vi "array_to_pixmap.vi"(11 "photoarray":u32[][](array[numeric])) -> (2 "pixmap out":T1, 3 "photoarray out":u32[][](array[numeric]))   [LabVIEW 2016]
uses:
  <vilib>/picture/picture.llb/imagedata.ctl
panel:
  out "new picture":picture
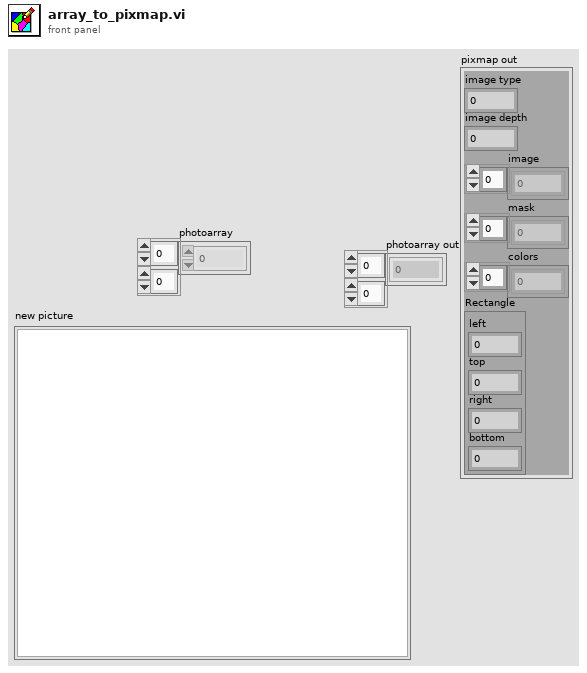
[diagram p1: front panel]
types:
  T1 = typedef "imagedata.ctl" = cluster{"image type":i32, "image depth":i32, "image":u8[], "mask":u8[], "colors":u32[], "Rectangle":cluster{"left":i16, "top":i16, "right":i16, "bottom":i16}}
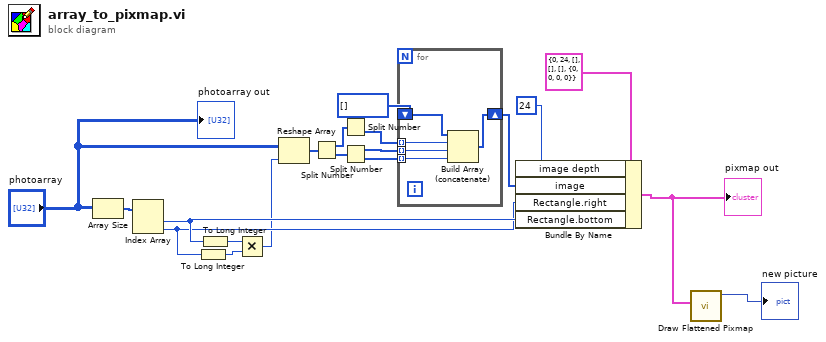
[diagram p0: block diagram]
diagram:
  n1 = Array Size(array="photoarray") -> (size(s)=w19:i32[])
  n2 = Index Array(array=w19) -> (element #1=w17:i32, element #2=w16:i32)  [unwired: 2 in]
  n3 = To Long Integer(number=w16) -> (32bit integer=w13:i32)
  n4 = To Long Integer(number=w17) -> (32bit integer=w14:i32)
  n5 = Multiply(x=w14, y=w13) -> (x*y=w12:i32)
  n6 = Reshape Array("photoarray", w12) -> (w11:u32[])
  n7 = Split Number(x=w11) -> (hi(x)=w10:u16[], lo(x)=w9:u16[])
  n8 = Split Number(x=w10) -> (lo(x)=w3:u8[])  [unwired: 1 out]
  n9 = Split Number(x=w9) -> (hi(x)=w4:u8[], lo(x)=w5:u8[])
  n10 = for {
    shift-right: [w24] -> w8
    shift-left: u8[] [] -> [w23]
    tunnel: w5 -> [w22] mode=indexing
    tunnel: w4 -> [w21] mode=indexing
    tunnel: w3 -> [w20] mode=indexing
    n11 = Build Array (concatenate)(w23, w20, w21, w22) -> (w24:u8[])
  }
  n12 = Bundle By Name(cluster=T1 {"image type"=0, "image depth"=24, "image"=[], "mask"=[], "colors"=[], "Rectangle"={"left"=0, "top"=0, "right"=0, "bottom"=0}} ("image data"), "image depth"=24, "image"=w8, "Rectangle.right"=w16, "Rectangle.bottom"=w17) -> (w2:T1)
  "pixmap out" <- w2
  n13 = call <vilib>:"Draw Flattened Pixmap.vi"("image data"=w2) -> ("new picture"=→"new picture":picture)  [unwired: 8 in]
  "photoarray out" <- "photoarray"
